vi "计算采集时间.vi"(6 "开始时间":string="090900", 7 "开始日期":string="20200805", 8 "时间间隔":string="100", 9 "重复次数":string="1", 10 "采样率":string="7", 11 "采样点数":string="40000") -> (0 "时间延迟":i32, 3 "采集时间":dbl)   [LabVIEW 2019]
panel:
  out "年数":i32
  out "月数":i32
  out "天数":i32
  out "小时数":i32
  out "分钟数":i32
  out "秒数":i32
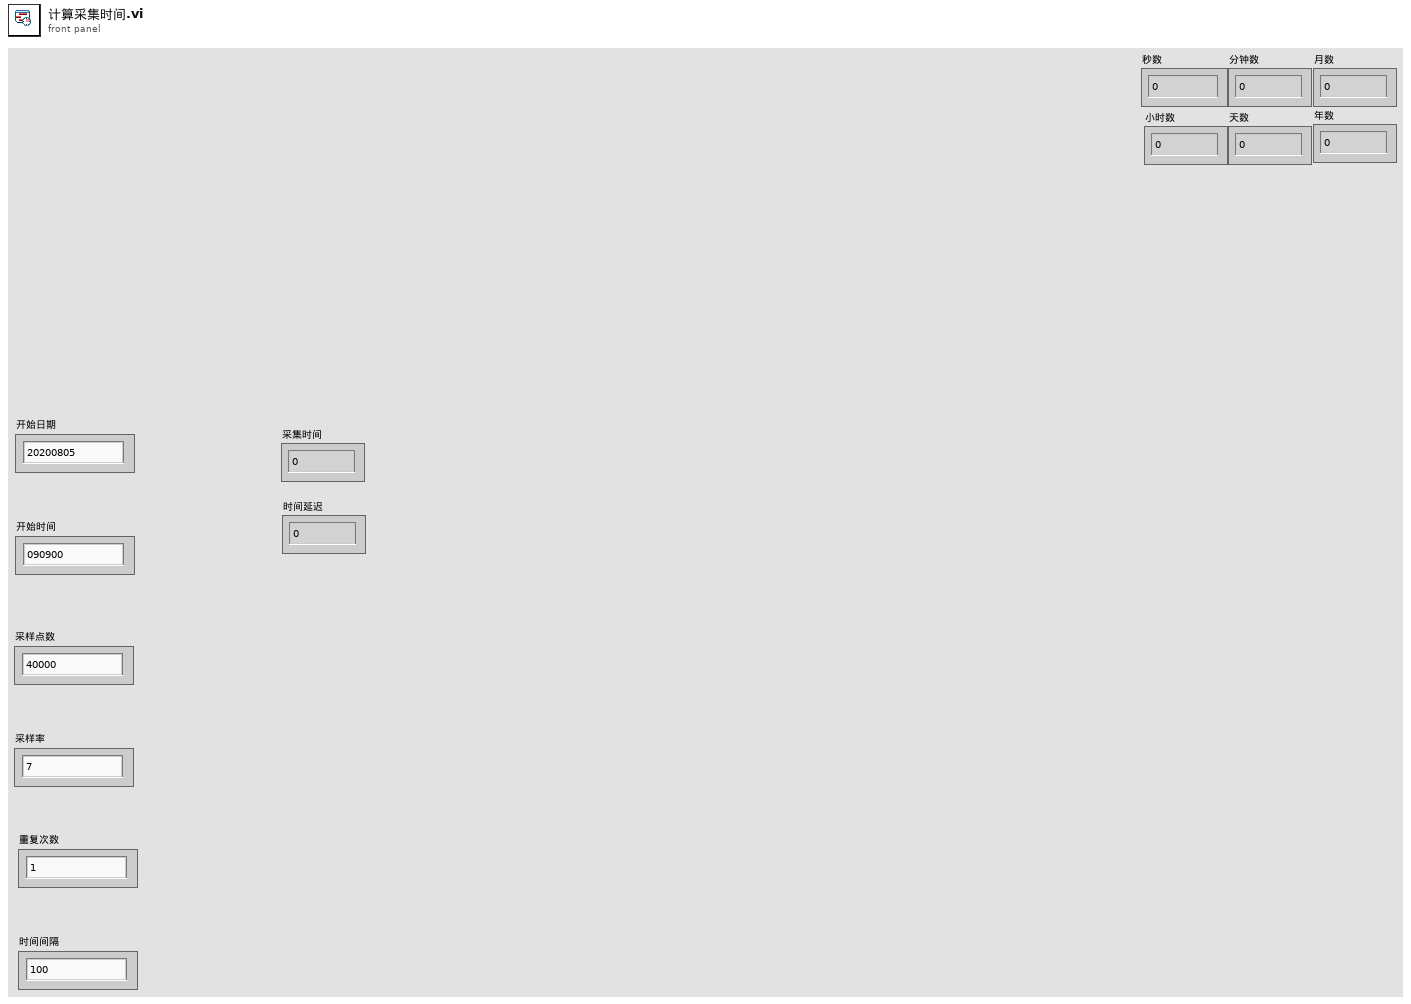
[diagram p1: front panel]
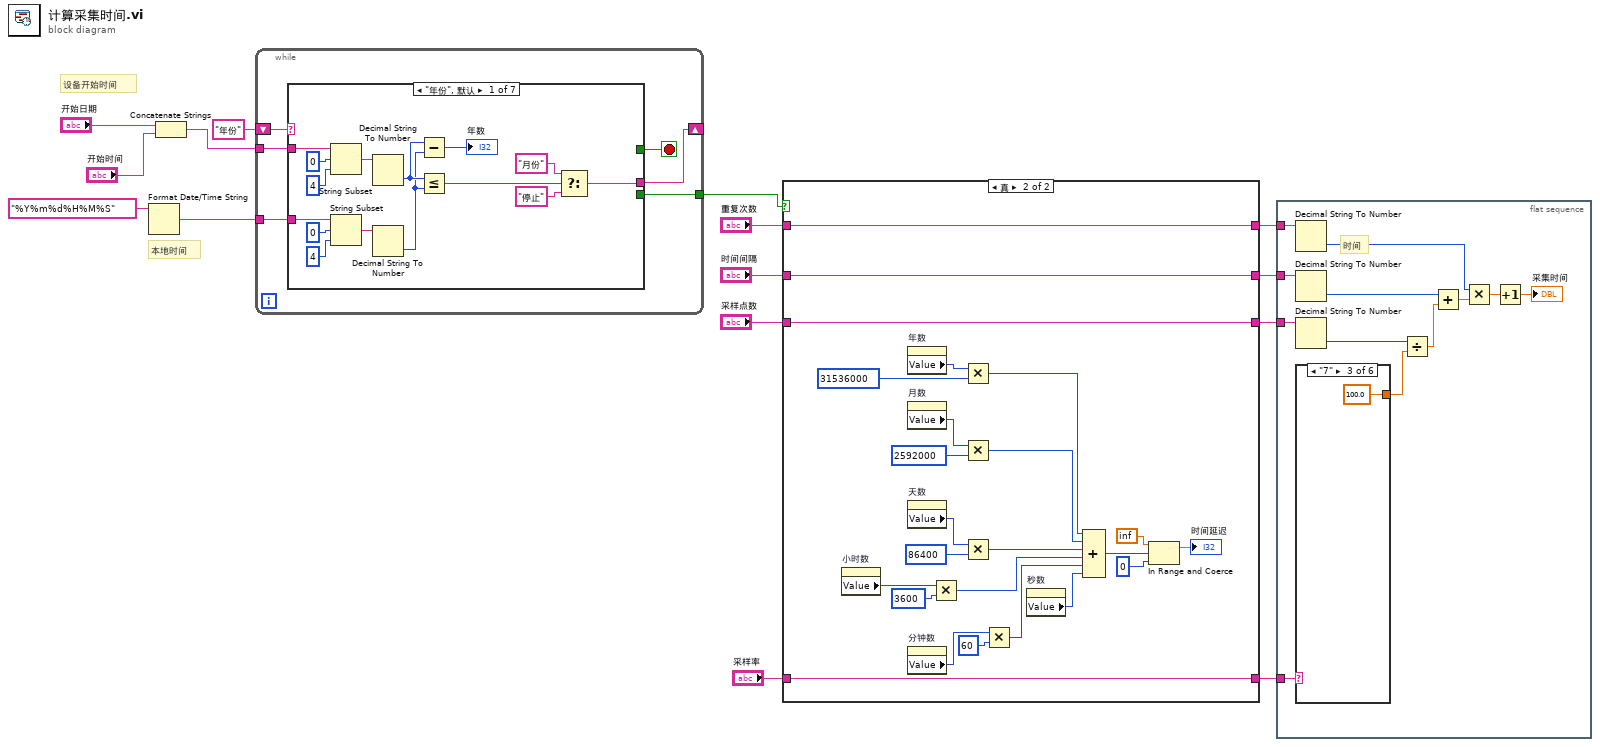
[diagram p0: block diagram]
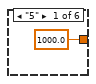
[diagram p2: hidden frame]
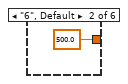
[diagram p3: hidden frame]
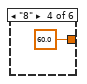
[diagram p4: hidden frame]
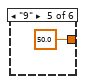
[diagram p5: hidden frame]
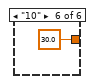
[diagram p6: hidden frame]
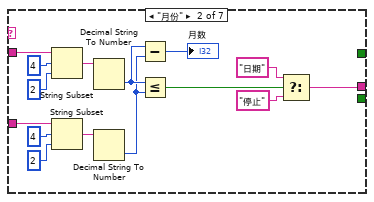
[diagram p7: hidden frame]
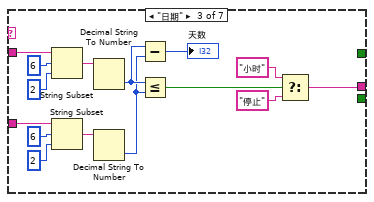
[diagram p8: hidden frame]
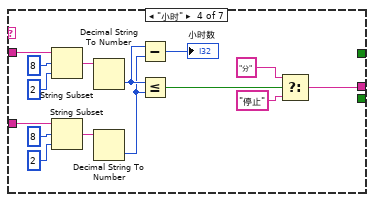
[diagram p9: hidden frame]
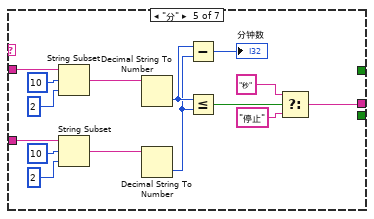
[diagram p10: hidden frame]
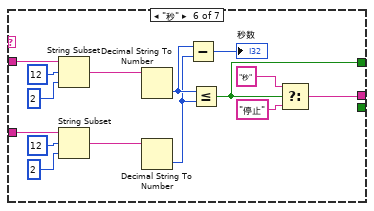
[diagram p11: hidden frame]
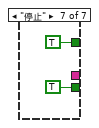
[diagram p12: hidden frame]
diagram:
  # "设备开始时间"
  # "本地时间"
  n1 = Format Date/Time String(time format string (%c)="%Y%m%d%H%M%S" ("时间格式字符串(%c)")) -> (date/time string=w13:string)  [unwired: 2 in]
  n2 = Concatenate Strings("开始日期", "开始时间") -> (w1:string)
  n3 = while {
    tunnel: w1 -> [w19]
    tunnel: w13 -> [w20]
    shift-right: [w18] -> _
    shift-left: "年份" -> [w21]
    tunnel: [w16] -> w2
    stop <- w17 stop-if-true
    n4 = case shown="\"年份\", 默认" w21 {
      tunnel: w19 -> [w36 w45 w59 w74 w89 w105 _]
      tunnel: w20 -> [w29 w44 w58 w73 w88 w104 _]
      tunnel: [w28 w43 w57 w72 w87 w102 _] -> w18
      tunnel: [_ _ _ _ _ w100 TRUE] -> w17
      tunnel: [_ _ _ _ _ _ TRUE] -> w16
      frame "年份", Default {
        n5 = String Subset(string=w36, offset (0)=0 ("偏移量(0)"), length (rest)=4 ("长度（剩余）")) -> (substring=w33:string)
        n6 = String Subset(string=w29, offset (0)=0 ("偏移量(0)"), length (rest)=4 ("长度（剩余）")) -> (substring=w32:string)
        n7 = Decimal String To Number(string=w33) -> (number=w24:i32)  [unwired: 2 in, 1 out]
        n8 = Decimal String To Number(string=w32) -> (number=w23:i32)  [unwired: 2 in, 1 out]
        n9 = Subtract(x=w24, y=w23) -> (x-y=→"年数":i32)
        n10 = Less Or Equal?(x=w24, y=w23) -> (x <= y?=w27:bool)
        n11 = Select(t="月份", s=w27, f="停止") -> (s? t:f=w28:string)
      }
      frame "月份" {
        n12 = String Subset(string=w45, offset (0)=4 ("偏移量(0)"), length (rest)=2 ("长度（剩余）")) -> (substring=w49:string)
        n13 = String Subset(string=w44, offset (0)=4 ("偏移量(0)"), length (rest)=2 ("长度（剩余）")) -> (substring=w48:string)
        n14 = Decimal String To Number(string=w49) -> (number=w39:i32)  [unwired: 2 in, 1 out]
        n15 = Decimal String To Number(string=w48) -> (number=w38:i32)  [unwired: 2 in, 1 out]
        n16 = Subtract(x=w39, y=w38) -> (x-y=→"月数":i32)
        n17 = Less Or Equal?(x=w39, y=w38) -> (x <= y?=w41:bool)
        n18 = Select(t="日期", s=w41, f="停止") -> (s? t:f=w43:string)
      }
      frame "日期" {
        n19 = String Subset(string=w59, offset (0)=6 ("偏移量(0)"), length (rest)=2 ("长度（剩余）")) -> (substring=w64:string)
        n20 = String Subset(string=w58, offset (0)=6 ("偏移量(0)"), length (rest)=2 ("长度（剩余）")) -> (substring=w63:string)
        n21 = Decimal String To Number(string=w64) -> (number=w54:i32)  [unwired: 2 in, 1 out]
        n22 = Decimal String To Number(string=w63) -> (number=w53:i32)  [unwired: 2 in, 1 out]
        n23 = Subtract(x=w54, y=w53) -> (x-y=→"天数":i32)
        n24 = Less Or Equal?(x=w54, y=w53) -> (x <= y?=w60:bool)
        n25 = Select(t="小时", s=w60, f="停止") -> (s? t:f=w57:string)
      }
      frame "小时" {
        n26 = String Subset(string=w74, offset (0)=8 ("偏移量(0)"), length (rest)=2 ("长度（剩余）")) -> (substring=w79:string)
        n27 = String Subset(string=w73, offset (0)=8 ("偏移量(0)"), length (rest)=2 ("长度（剩余）")) -> (substring=w78:string)
        n28 = Decimal String To Number(string=w79) -> (number=w69:i32)  [unwired: 2 in, 1 out]
        n29 = Decimal String To Number(string=w78) -> (number=w68:i32)  [unwired: 2 in, 1 out]
        n30 = Subtract(x=w69, y=w68) -> (x-y=→"小时数":i32)
        n31 = Less Or Equal?(x=w69, y=w68) -> (x <= y?=w75:bool)
        n32 = Select(t="分", s=w75, f="停止") -> (s? t:f=w72:string)
      }
      frame "分" {
        n33 = String Subset(string=w89, offset (0)=10 ("偏移量(0)"), length (rest)=2 ("长度（剩余）")) -> (substring=w94:string)
        n34 = String Subset(string=w88, offset (0)=10 ("偏移量(0)"), length (rest)=2 ("长度（剩余）")) -> (substring=w93:string)
        n35 = Decimal String To Number(string=w94) -> (number=w84:i32)  [unwired: 2 in, 1 out]
        n36 = Decimal String To Number(string=w93) -> (number=w83:i32)  [unwired: 2 in, 1 out]
        n37 = Subtract(x=w84, y=w83) -> (x-y=→"分钟数":i32)
        n38 = Less Or Equal?(x=w84, y=w83) -> (x <= y?=w90:bool)
        n39 = Select(t="秒", s=w90, f="停止") -> (s? t:f=w87:string)
      }
      frame "秒" {
        n40 = String Subset(string=w105, offset (0)=12 ("偏移量(0)"), length (rest)=2 ("长度（剩余）")) -> (substring=w109:string)
        n41 = String Subset(string=w104, offset (0)=12 ("偏移量(0)"), length (rest)=2 ("长度（剩余）")) -> (substring=w108:string)
        n42 = Decimal String To Number(string=w109) -> (number=w99:i32)  [unwired: 2 in, 1 out]
        n43 = Decimal String To Number(string=w108) -> (number=w98:i32)  [unwired: 2 in, 1 out]
        n44 = Subtract(x=w99, y=w98) -> (x-y=→"秒数":i32)
        n45 = Less Or Equal?(x=w99, y=w98) -> (x <= y?=w100:bool)
        n46 = Select(t="秒", s=w100, f="停止") -> (s? t:f=w102:string)
      }
      frame "停止" {
      }
    }
  }
  n47 = case shown="真" w2 {
    tunnel: "时间间隔" -> [w117 w141]
    tunnel: [w117 w141] -> w9
    tunnel: [w116 w140] -> w8
    tunnel: "采样率" -> [w116 w140]
    tunnel: "采样点数" -> [w115 w139]
    tunnel: [w115 w139] -> w5
    tunnel: "重复次数" -> [w114 w138]
    tunnel: [w114 w138] -> w3
    frame False {
    }
    frame True {
      n48 = property on="小时数" class="DigNum (严格)"() -> ("Value"=w131:i32)  [unwired: 2 in, 2 out]
      n49 = property on="年数" class="DigNum (严格)"() -> ("Value"=w137:i32)  [unwired: 2 in, 2 out]
      n50 = property on="月数" class="DigNum (严格)"() -> ("Value"=w135:i32)  [unwired: 2 in, 2 out]
      n51 = property on="天数" class="DigNum (严格)"() -> ("Value"=w133:i32)  [unwired: 2 in, 2 out]
      n52 = property on="分钟数" class="DigNum (严格)"() -> ("Value"=w128:i32)  [unwired: 2 in, 2 out]
      n53 = Multiply(x=w131, y=3600) -> (x*y=w124:i32)
      n54 = Multiply(x=w137, y=31536000) -> (x*y=w127:i32)
      n55 = Multiply(x=w135, y=2592000) -> (x*y=w126:i32)
      n56 = Multiply(x=w133, y=86400) -> (x*y=w125:i32)
      n57 = Multiply(x=w128, y=60) -> (x*y=w123:i32)
      n58 = property on="秒数" class="DigNum (严格)"() -> ("Value"=w122:i32)  [unwired: 2 in, 2 out]
      n59 = Compound Arithmetic op=ADD(w127, w126, w125, w124, w123, w122) -> (w121:i32)
      n60 = In Range and Coerce(upper limit=inf, x=w121, lower limit=0 ("下限")) -> (coerced(x)=→"时间延迟":dbl)  [unwired: 1 out]
    }
  }
  n61 = flat-sequence {
    tunnel: w9 -> [w145]
    tunnel: w8 -> [w144]
    tunnel: w5 -> [w143]
    tunnel: w3 -> [w142]
    frame #0 {
      # "时间"
      n62 = Decimal String To Number(string=w142) -> (number=w148:i32)  [unwired: 2 in, 1 out]
      n63 = Decimal String To Number(string=w145) -> (number=w149:i32)  [unwired: 2 in, 1 out]
      n64 = Decimal String To Number(string=w143) -> (number=w146:i32)  [unwired: 2 in, 1 out]
      n65 = case shown="\"7\"" w144 {
        tunnel: [1000.0 ("进度条") 500.0 ("进度条") 100.0 ("进度条") 60.0 ("进度条") 50.0 ("进度条") 30.0 ("进度条")] -> w147
        frame "5" {
        }
        frame "6", Default {
        }
        frame "7" {
        }
        frame "8" {
        }
        frame "9" {
        }
        frame "10" {
        }
      }
      n66 = Divide(x=w146, y=w147) -> (x/y=w151:dbl)
      n67 = Add(x=w149, y=w151) -> (x+y=w150:dbl)
      n68 = Multiply(x=w148, y=w150) -> (x*y=w152:dbl)
      n69 = Increment(x=w152) -> (x+1=→"采集时间":dbl)
    }
  }
